vi "SRV_Queue_Enqueue Element.vi"(6 "timeout in ms (-1)":i32, 8 "error in (no error)":errorcluster, 9 "Data":variant, 10 "Command":string, 11 "Command-Data Queue":refnum<queue>) -> (0 "error out":errorcluster, 1 "timed out?":bool, 3 "Command-Data Queue out":refnum<queue>)   [LabVIEW 2014]
doc: "Enqueues an element onto the referenced Command-Data Queue.\n\n\nAuthor: Mike Schultz - Logic PD"
uses:
  SRV_Command-Data Queue Data Type.ctl
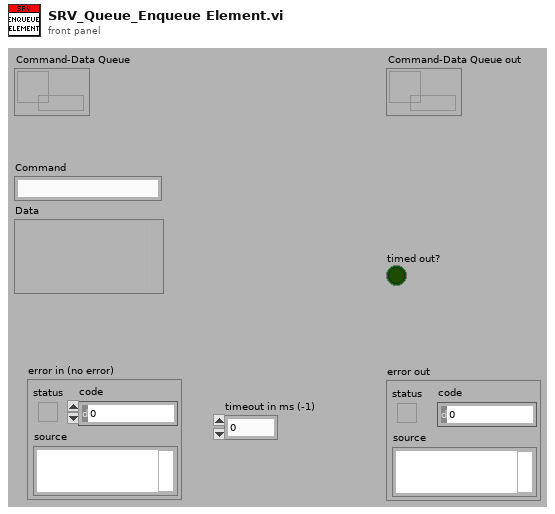
[diagram p1: front panel]
types:
  T1 = typedef "SRV_Command-Data Queue Data Type.ctl" = cluster{"Command":string, "Data":variant}
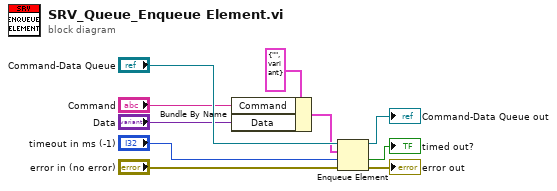
[diagram p0: block diagram]
diagram:
  n1 = Bundle By Name(cluster=T1 {"Command"="", "Data"=variant} ("Queue Data Type"), "Command"="Command", "Data"="Data") -> (w3:T1)
  n2 = Enqueue Element(queue="Command-Data Queue", element=w3, timeout in ms (-1)="timeout in ms (-1)", error in (no error)="error in (no error)") -> (queue out=→"Command-Data Queue out":refnum<queue>, timed out?=→"timed out?":bool, error out=→"error out":errorcluster)
